vi "Set-ControlSignal.vi"(3 "error in (no error)":errorcluster, 4 "Voltage / Volts":dbl min=-15.0 max=15.0, 5 "Output channel":T1, 6 "VISA resource name":refnum<visa-resource-name>) -> (0 "error out":errorcluster, 2 "VISA resource name out":refnum<visa-resource-name>)   [LabVIEW 2014, in "YbTempCtrl.lvlib"]
doc: "Manually set the output of the device to the given value. This will not affect the setpoint of the lock if the device is locking."
uses:
  YbTempCtrl.lvlib
  Typedefs/OutputChannelTypedef.ctl
panel:
  out "Config string":string
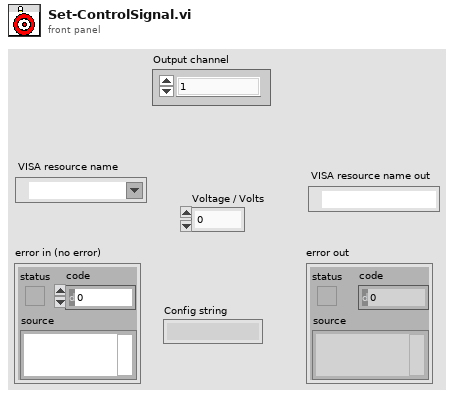
[diagram p1: front panel]
types:
  T1 = typedef "YbTempCtrl.lvlib/OutputChannelTypedef.ctl" = enum16{"1", "2", "3", "4", "BPA", "BPB"}
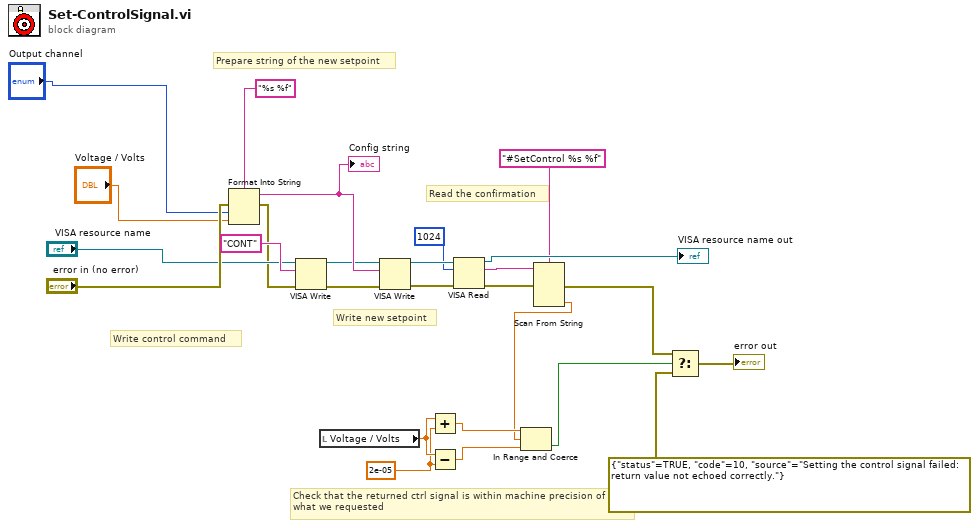
[diagram p0: block diagram]
diagram:
  w20 = 2e-05
  # "Check that the returned ctrl signal is within machine precision of\nwhat we requested"
  # "Read the confirmation"
  # "Write new setpoint"
  # "Prepare string of the new setpoint"
  # "Write control command"
  n1 = Format Into String(format string="%s %f", error in="error in (no error)", "Output channel", "Voltage / Volts") -> (resulting string=w25:string, error out=w12:errorcluster)  [unwired: 1 in]
  "Config string" <- w25
  n2 = VISA Write(VISA resource name="VISA resource name", write buffer="CONT", error in (no error)=w12) -> (VISA resource name out=w14:refnum<visa-resource-name>, error out=w13:errorcluster)  [unwired: 1 out]
  n3 = local read "Voltage / Volts"() -> (w21:dbl)
  n4 = VISA Write(VISA resource name=w14, write buffer=w25, error in (no error)=w13) -> (VISA resource name out=w24:refnum<visa-resource-name>, error out=w23:errorcluster)  [unwired: 1 out]
  n5 = Add(x=w21, y=w20) -> (x+y=w6:dbl)
  n6 = Subtract(x=w21, y=w20) -> (x-y=w5:dbl)
  n7 = VISA Read(VISA resource name=w24, byte count=u32 1024, error in (no error)=w23) -> (VISA resource name out=→"VISA resource name out":refnum<visa-resource-name>, read buffer=w10:string, error out=w8:errorcluster)  [unwired: 1 out]
  n8 = Scan From String(format string="#SetControl %s %f", input string=w10, error in=w8) -> (error out=w7:errorcluster, output 2=w2:dbl)  [unwired: 4 in, 2 out]
  n9 = In Range and Coerce(upper limit=w6, x=w2, lower limit=w5) -> (In Range?=w3:bool)  [unwired: 1 out]
  n10 = Select(t=w7, s=w3, f=errorcluster {"status"=TRUE, "code"=10, "source"="Setting the control signal failed: return value not echoed correctly."}) -> (s? t:f=→"error out":errorcluster)
